vi "Main Test Panel.vi"() -> ()   [LabVIEW 2013]
uses:
  Controls/DAQ Cluster.ctl
  <vilib>/DAQmx/create/channels.llb/DAQmx Create Channel (AI-Voltage-Basic).vi
panel:
  in  "Daq Clust 2":T2={"Save"=FALSE, "DAQ Cluster"={"PSI Channel"="Dev1/ai9", "TC Channel"="Dev1/ai10", "PSI Offset"=0.555, "PSI Scale"=3000.0, "TC Offset"=1.028, "TC Scale"=144.0}, "Cancel"=FALSE}
  in  "Start Averaging":bool
  in  "Time and Date":string
  out "DAQ On?":bool
  in  "Sim Cluster":T3 {"Temp" scale=0.0..35.0; "PSI" scale=0.0..20000.0}
  in  "Print to PDF":bool
  in  "Clear Graph":bool
  in  "DAQ Stop":bool
  in  "DAQ Start":bool
  in  "Test Duration (mins)":i32
  in  "Pressure (PSI)":i32
  in  "Test Temperature (°C)":i32
  in  "Tech Initials":string
  in  "Customer":string
  in  "Proof Test\nPressure (PSI)":i32
  in  "Time @ Proof\nPressure (mins)":i32=30
  in  "Max Working\nPressure (PSI)":i32
  in  "Serial #":string
  in  "Part Desc.":string
  in  "Part #":string
  out "Pressure Graph":dbl[][](graph)
  in  "Test Result":string
  # "Pressure Certificate"
  # "982 North 675 West\nNorth Salt Lake, UT 84054"
  # "Test Information"
  # "Test Results"
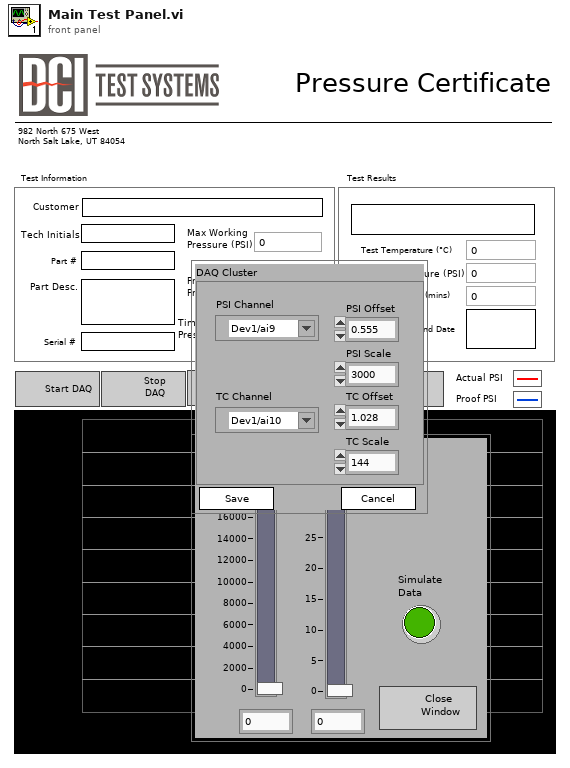
[diagram p1: front panel]
types:
  T1 = typedef "DAQ Cluster.ctl" = cluster{"PSI Channel":tag, "TC Channel":tag, "PSI Offset":dbl, "PSI Scale":dbl, "TC Offset":dbl, "TC Scale":dbl}
  T2 = cluster{"Save":bool, "DAQ Cluster":T1, "Cancel":bool}
  T3 = cluster{"PSI":i32, "Temp":i32, "Simulate\nData":bool, "Close Sim":bool}
  T4 = enum16{"open", "replace", "create", "open or create", "replace or create", "replace or create with confirmation"}
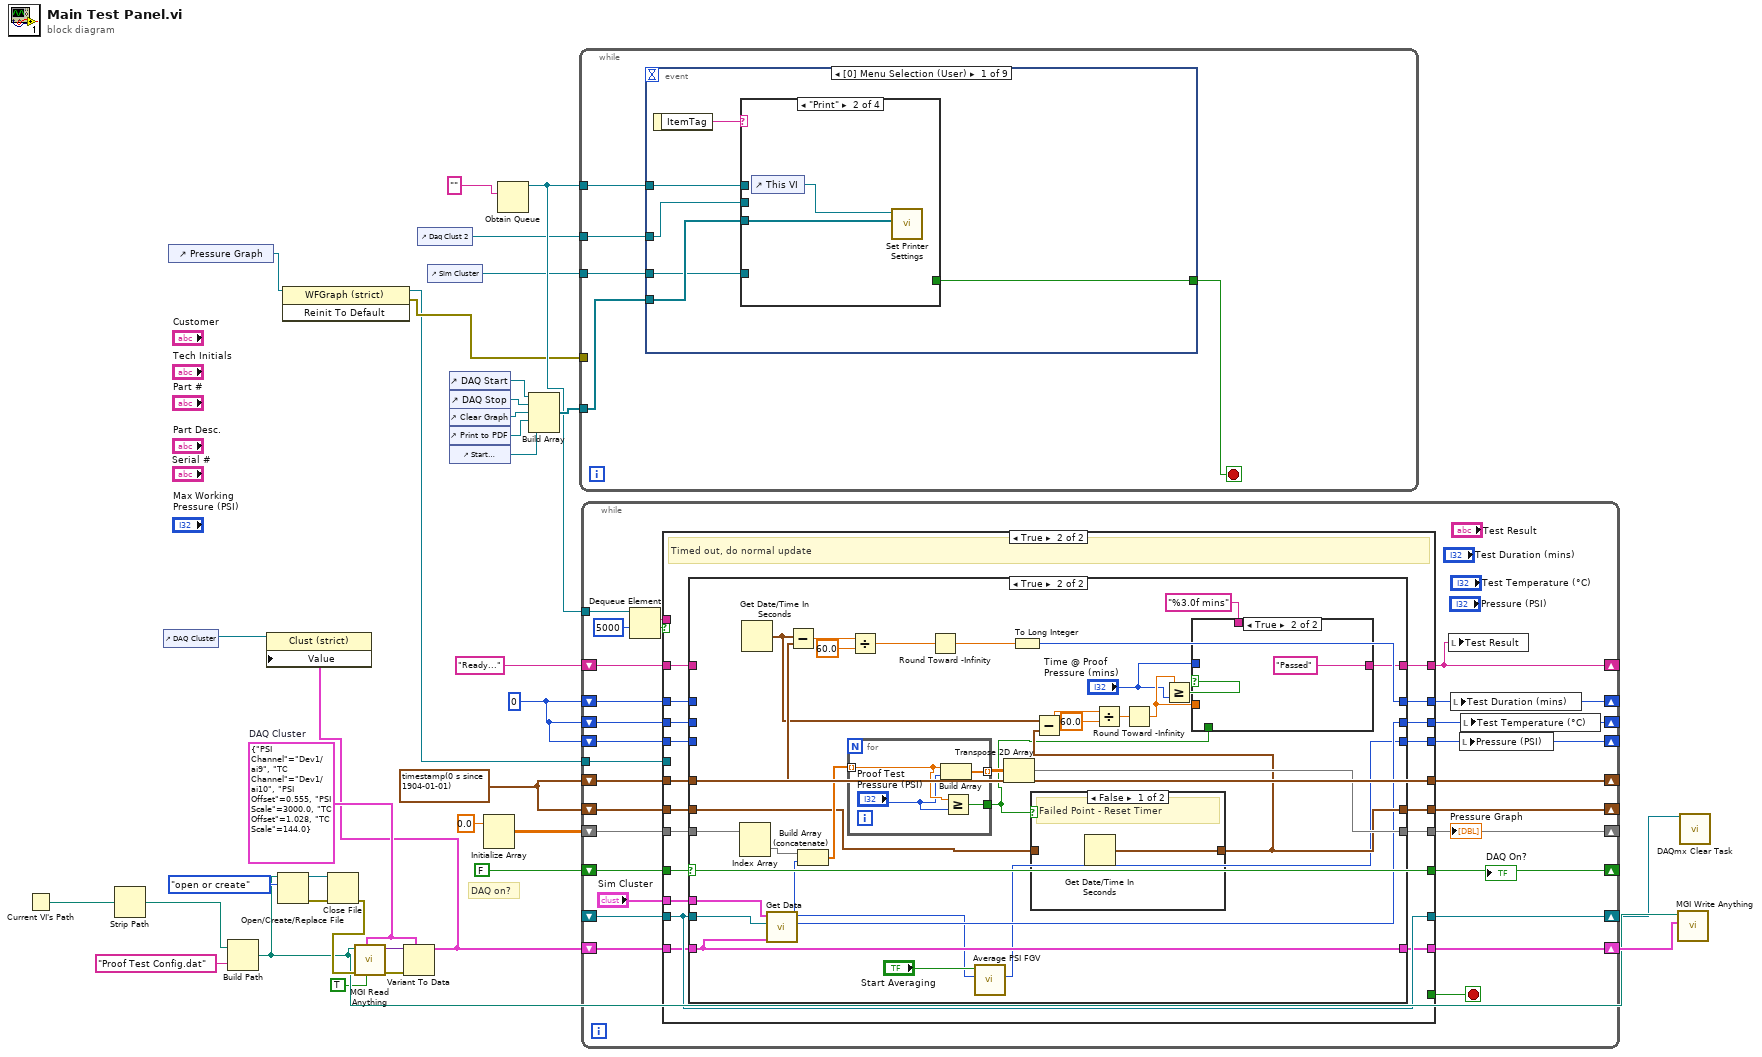
[diagram p0: block diagram]
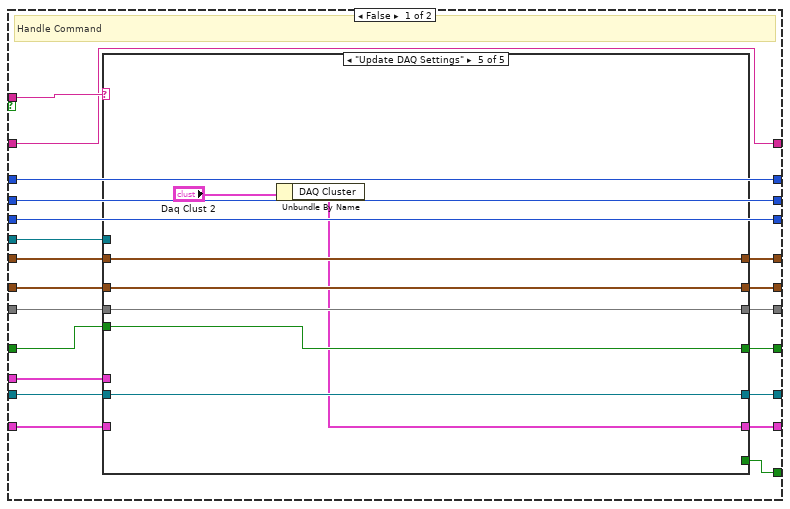
[diagram p2: hidden frame]
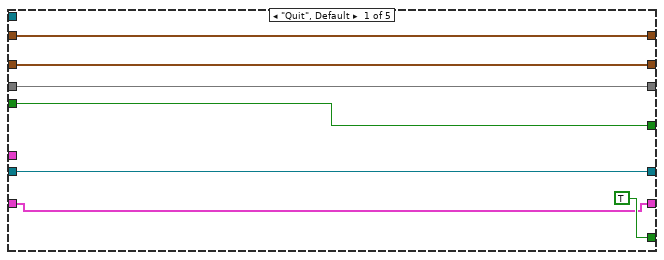
[diagram p3: hidden frame]
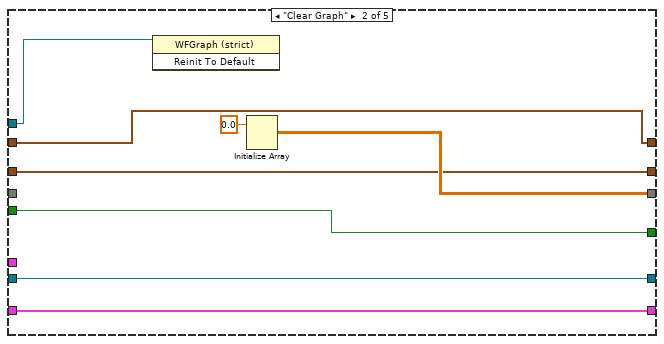
[diagram p4: hidden frame]
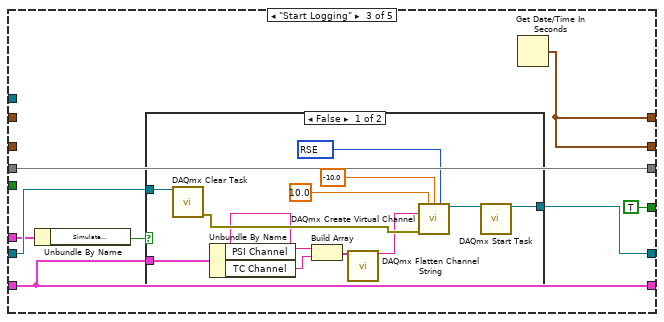
[diagram p5: hidden frame]
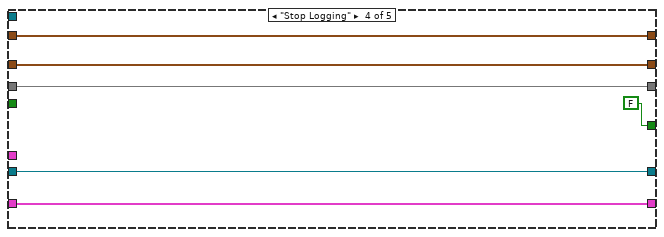
[diagram p7: hidden frame]
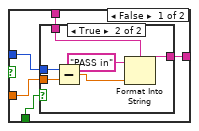
[diagram p9: hidden frame]
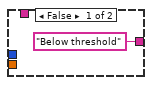
[diagram p10: hidden frame]
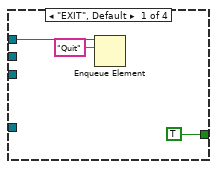
[diagram p12: hidden frame]
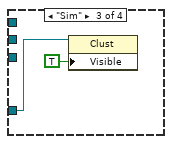
[diagram p13: hidden frame]
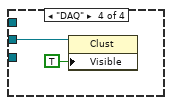
[diagram p14: hidden frame]
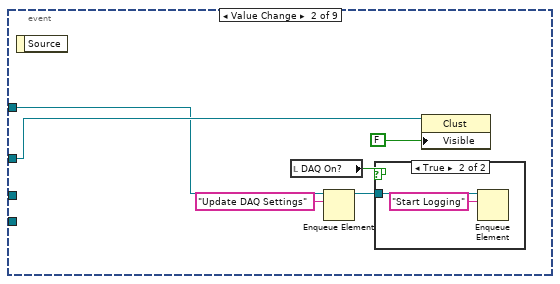
[diagram p15: hidden frame]
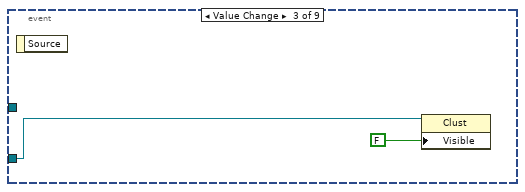
[diagram p17: hidden frame]
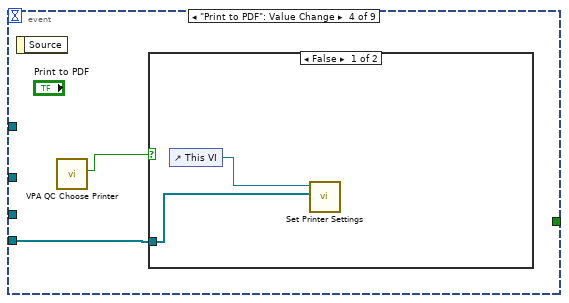
[diagram p18: hidden frame]
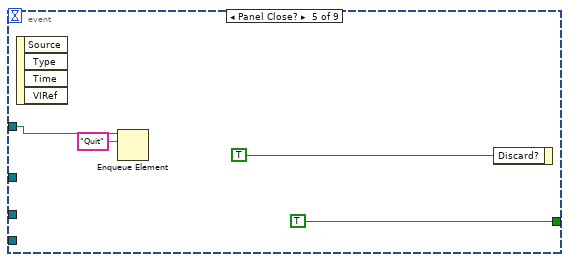
[diagram p20: hidden frame]
diagram:
  w10 = T1 {"PSI Channel"="Dev1/ai9", "TC Channel"="Dev1/ai10", "PSI Offset"=0.555, "PSI Scale"=3000.0, "TC Offset"=1.028, "TC Scale"=144.0}  # DAQ Cluster
  w21 = timestamp(0 s since 1904-01-01)
  w23 = 0 ("Test Duration (mins)")
  # "DAQ on?"
  n1 = Current VI's Path() -> (path=w16:path)
  n2 = Strip Path(path=w16) -> (stripped path=w5:path)  [unwired: 1 out]
  n3 = control-ref of="DAQ Cluster"() -> (w4:refnum<vi>)
  n4 = control-ref of="Pressure Graph"() -> (w28:refnum<vi>)
  n5 = Build Path(base path=w5, name or relative path="Proof Test Config.dat") -> (appended path=w8:path)
  n6 = Open/Create/Replace File(file path (use dialog)=w8, operation (0:open)=T4."open or create") -> (refnum out=w13:refnum<file>, error out=w12:errorcluster)  [unwired: 4 in, 1 out]
  n7 = invoke class="WFGraph (strict)" method="Reinit To Default"(reference=w28) -> (reference out=w19:refnum<vi>, error out=w25:errorcluster)  [unwired: 2 in, 1 out]
  n8 = Close File(refnum=w13, error in=w12) -> (error out=w11:errorcluster)  [unwired: 1 out]
  n9 = call <userlib>:"MGI Read Anything.vi"("Use Supplied (F: Use Default)"=TRUE, "Type of Anything"=w10, "Error In"=w11, "Path (dialog)"=w8) -> ("Error Out"=w18:errorcluster, "Anything"=w17:variant)  [unwired: 4 in, 2 out]
  n10 = Variant To Data(error in=w18, type=w10, Variant=w17) -> (data=w3:T1)  [unwired: 1 out]
  n11 = property class="Clust (strict)"(reference=w4, "Value"=w3) -> ()  [unwired: 1 in, 2 out]
  n12 = control-ref of="Daq Clust 2"() -> (w6:refnum<vi>)
  n13 = control-ref of="Sim Cluster"() -> (w20:refnum<vi>)
  n14 = control-ref of="DAQ Start"() -> (w35:refnum<vi>)
  n15 = control-ref of="DAQ Stop"() -> (w34:refnum<vi>)
  n16 = control-ref of="Clear Graph"() -> (w33:refnum<vi>)
  n17 = control-ref of="Print to PDF"() -> (w32:refnum<vi>)
  n18 = control-ref of="Start Averaging"() -> (w1:refnum<vi>)
  n19 = Initialize Array(0.0 ("element")) -> (w26:dbl[][])  [unwired: 2 in]
  n20 = Obtain Queue(element data type="") -> (queue out=w30:refnum<queue>)  [unwired: 4 in, 2 out]
  n21 = Build Array(w35, w34, w33, w32, w1) -> (w31:refnum<vi>[])
  n22 = while {
    tunnel: w31 -> [w39]
    tunnel: w30 -> [w38]
    tunnel: w25 -> [_]
    tunnel: w20 -> [w37]
    tunnel: w6 -> [w36]
    stop <- w40 stop-if-true
    n23 = event shown="[0] Menu Selection (User)" {
      selector: _ -> [_ _ _ _ _ _ _ _ _]
      dyn-events: _ -> [_ _ _ _ _ _ _ _ _]
      timeout: _ -> [_ _ _ _ _ _ _ _ _]
      tunnel: [w45 _ _ _ TRUE _ _ _ _] -> w40
      tunnel: w39 -> [w44 _ _ w66 _ _ _ _ _]
      tunnel: w38 -> [w43 w59 _ _ w71 w75 w82 w84 _]
      tunnel: w37 -> [w42 _ _ _ _ _ _ _ w86]
      tunnel: w36 -> [w41 w61 w65 _ _ _ _ _ _]
      event Menu Selection (User) {
        n24 = event-data() -> ("ItemTag"=w46:string)  [unwired: 1 in]
        n25 = case shown="\"Print\"" w46 {
          tunnel: [TRUE _ _ _] -> w45
          tunnel: w44 -> [_ w50 _ _]
          tunnel: w43 -> [w48 _ _ _]
          tunnel: w42 -> [_ _ w53 _]
          tunnel: w41 -> [_ _ _ w54]
          frame "EXIT", Default {
            n26 = Enqueue Element(queue=w48, element="Quit") -> ()  [unwired: 2 in, 3 out]
          }
          frame "Print" {
            n27 = control-ref of="This VI"() -> (w51:refnum<vi>)
            n28 = call "Set Printer Settings.vi"("Array"=w50, "VI in"=w51) -> ()  [unwired: 10 in]
          }
          frame "Sim" {
            n29 = property class="Clust"(reference=w53, "Visible"=TRUE) -> ()  [unwired: 1 in, 2 out]
          }
          frame "DAQ" {
            n30 = property class="Clust"(reference=w54, "Visible"=TRUE) -> ()  [unwired: 1 in, 2 out]
          }
        }
      }
      event "Daq Clust 2.Save": Value Change {
        n31 = event-data() -> ()  [unwired: 1 in, 1 out]
        n32 = local read "DAQ On?"() -> (w56:bool)
        n33 = Enqueue Element(queue=w59, element="Update DAQ Settings") -> (queue out=w57:refnum<queue>)  [unwired: 2 in, 2 out]
        n34 = case shown="True" w56 {
          tunnel: w57 -> [_ w63]
          frame False {
          }
          frame True {
            n35 = Enqueue Element(queue=w63, element="Start Logging") -> ()  [unwired: 2 in, 3 out]
          }
        }
        n36 = property class="Clust"(reference=w61, "Visible"=FALSE) -> ()  [unwired: 1 in, 2 out]
      }
      event "Daq Clust 2.Cancel": Value Change {
        n37 = event-data() -> ()  [unwired: 1 in, 1 out]
        n38 = property class="Clust"(reference=w65, "Visible"=FALSE) -> ()  [unwired: 1 in, 2 out]
      }
      event "Print to PDF": Value Change {
        n39 = event-data() -> ()  [unwired: 1 in, 1 out]
        n40 = call "VPA QC Choose Printer.vi"() -> ("Cancelled"=w67:bool)  [unwired: 11 in]
        n41 = case shown="False" w67 {
          tunnel: w66 -> [w69 _]
          frame False {
            n42 = control-ref of="This VI"() -> (w68:refnum<vi>)
            n43 = call "Set Printer Settings.vi"("Array"=w69, "VI in"=w68) -> ()  [unwired: 10 in]
          }
          frame True {
          }
        }
      }
      event Panel Close? {
        n44 = event-data() -> ()  [unwired: 1 in, 4 out]
        n45 = Enqueue Element(queue=w71, element="Quit") -> ()  [unwired: 2 in, 3 out]
        n46 = event-data("Discard?"=TRUE) -> ()  [unwired: 1 in, 1 out]
      }
      event "Clear Graph": Value Change {
        n47 = event-data() -> ()  [unwired: 1 in, 1 out]
        n48 = Enqueue Element(queue=w75, element="Clear Graph") -> ()  [unwired: 2 in, 3 out]
      }
      event "DAQ Start": Value Change {
        n49 = event-data() -> ()  [unwired: 1 in, 1 out]
        n50 = Enqueue Element(queue=w82, element="Start Logging") -> ()  [unwired: 2 in, 3 out]
        n51 = Get Date/Time In Seconds() -> (seconds since 1Jan1904=w80:timestamp)
        n52 = Get Date/Time String(seconds (now)=w80) -> (date string=w77:string, time string=w79:string)  [unwired: 2 in]
        n53 = Concatenate Strings(w79, "\n" ("string"), w77) -> (w76:string)
        n54 = local write "Time and Date"(w76) -> ()
      }
      event "DAQ Stop": Value Change {
        n55 = event-data() -> ()  [unwired: 1 in, 1 out]
        n56 = Enqueue Element(queue=w84, element="Stop Logging") -> ()  [unwired: 2 in, 3 out]
      }
      event "Sim Cluster.Close Sim": Value Change {
        n57 = event-data() -> ()  [unwired: 1 in, 6 out]
        n58 = property class="Clust"(reference=w86, "Visible"=FALSE) -> ()  [unwired: 1 in, 2 out]
      }
    }
  }
  n59 = while {
    tunnel: w30 -> [w113]
    shift-right: [w105] -> _
    shift-left: w26 -> [w108]
    shift-right: [w106] -> _
    shift-left: FALSE -> [w107]
    shift-right: [w91] -> _
    shift-left: "Ready..." -> [w104]
    shift-right: [w89] -> _
    shift-left: w23 -> [w103]
    shift-right: [w90] -> _
    shift-left: w23 -> [w102]
    shift-right: [w88] -> _
    shift-left: w23 -> [w101]
    shift-right: [w100] -> _
    shift-left: w21 -> [w99]
    shift-right: [w97] -> _
    shift-left: w21 -> [w98]
    tunnel: w19 -> [w96]
    shift-right: [w95] -> w2
    shift-left: _ -> [w94]
    shift-right: [w92] -> w9
    shift-left: w3 -> [w93]
    stop <- w109 stop-if-true
    n60 = Dequeue Element(queue=w113, timeout in ms (-1)=5000) -> (element=w110:string, timed out?=w112:bool)  [unwired: 1 in, 2 out]
    n61 = case shown="True" w112 {
      tunnel: w110 -> [w133 _]
      tunnel: [w132 _] -> w109
      tunnel: w108 -> [w131 w197]
      tunnel: [w130 w195] -> w105
      tunnel: w107 -> [w129 w194]
      tunnel: [w128 w194] -> w106
      tunnel: w104 -> [w127 w190]
      tunnel: [w127 w188] -> w91
      tunnel: [w124 w199] -> w89
      tunnel: w103 -> [w124 w193]
      tunnel: [w123 w198] -> w90
      tunnel: w102 -> [w123 w191]
      tunnel: [w122 w196] -> w88
      tunnel: w101 -> [w122 w192]
      tunnel: [w126 w200] -> w100
      tunnel: w99 -> [w125 w200]
      tunnel: w98 -> [w120 w189]
      tunnel: [w121 w187] -> w97
      tunnel: w96 -> [w119 _]
      tunnel: [w118 w186] -> w95
      tunnel: w94 -> [w117 w186]
      tunnel: w93 -> [w116 w185]
      tunnel: [w115 w184] -> w92
      tunnel: "Sim Cluster" -> [w114 w183]
      frame False {
        # "Handle Command"
        n62 = case shown="\"Update DAQ Settings\"" w133 {
          tunnel: [TRUE _ _ _ _] -> w132
          tunnel: w131 -> [w139 _ w156 w175 w178]
          tunnel: w119 -> [_ w147 _ _ _]
          tunnel: [w139 w146 w156 w175 w178] -> w130
          tunnel: w129 -> [w138 w145 _ _ w179]
          tunnel: [w138 w145 TRUE FALSE w179] -> w128
          tunnel: [w137 w144 w154 w173 w182] -> w126
          tunnel: w125 -> [w137 w144 _ w173 w182]
          tunnel: [w136 w143 w154 w172 w181] -> w121
          tunnel: w120 -> [w136 w143 _ w172 w181]
          tunnel: [w135 w142 w151 w171 w180] -> w118
          tunnel: w117 -> [w135 w142 w152 w171 w180]
          tunnel: w116 -> [w134 w141 w153 w170 _]
          tunnel: [w134 w141 w153 w170 w176] -> w115
          tunnel: w114 -> [_ _ w150 _ _]
          frame "Quit", Default {
          }
          frame "Clear Graph" {
            n63 = invoke class="WFGraph (strict)" method="Reinit To Default"(reference=w147) -> ()  [unwired: 2 in, 3 out]
            n64 = Initialize Array(0.0 ("element")) -> (w146:dbl[][])  [unwired: 2 in]
          }
          frame "Start Logging" {
            n65 = Unbundle By Name(w150) -> ("Simulate\nData"=w149:bool)
            n66 = case shown="False" w149 {
              tunnel: w153 -> [w165 _]
              tunnel: w152 -> [w163 w169]
              tunnel: [w161 w169] -> w151
              frame False {
                w168 = 10083 items=["default"=-1, "RSE"=10083, "NRSE"=10078, "Differential"=10106, "Pseudodifferential"=12529] ("input terminal configuration")
                n67 = call <vilib>:"DAQmx Clear Task.vi"("task in"=w163) -> ("error out"=w162:errorcluster)  [unwired: 14 in]
                n68 = Unbundle By Name(w165) -> ("PSI Channel"=w160:tag, "TC Channel"=w159:tag)
                n69 = Build Array(w160, w159) -> (w158:tag[])
                n70 = call <vilib>:"DAQmx Flatten Channel String.vi"("names in"=w158) -> ("names out"=w157:string)  [unwired: 13 in, 1 out]
                n71 = call-poly <vilib>:"DAQmx Create Virtual Channel.vi"("maximum value"=10.0, "minimum value"=-10.0, "input terminal configuration"=w168, "physical channels"=w157, "error in"=w162) -> ("task out"=w164:refnum<k21>)  [unwired: 9 in, 1 out]
                n72 = call <vilib>:"DAQmx Start Task.vi"("task/channels in"=w164) -> ("task out"=w161:refnum<k21>)  [unwired: 13 in, 1 out]
              }
              frame True {
              }
            }
            n73 = Get Date/Time In Seconds() -> (seconds since 1Jan1904=w154:timestamp)
          }
          frame "Stop Logging" {
          }
          frame "Update DAQ Settings" {
            n74 = Unbundle By Name("Daq Clust 2") -> ("DAQ Cluster"=w176:T1)
          }
        }
      }
      frame True {
        # "Timed out, do normal update"
        n75 = case shown="True" w194 {
          tunnel: w200 -> [_ w237]
          tunnel: [w207 w233] -> w199
          tunnel: [w204 w214] -> w198
          tunnel: w197 -> [w206 w232]
          tunnel: [w205 w210] -> w196
          tunnel: [w206 w228] -> w195
          tunnel: w193 -> [w207 _]
          tunnel: w192 -> [w205 _]
          tunnel: w191 -> [w204 _]
          tunnel: w190 -> [w203 _]
          tunnel: w189 -> [w202 w226]
          tunnel: [w203 w220] -> w188
          tunnel: [w202 w219] -> w187
          tunnel: w186 -> [_ w213]
          tunnel: w185 -> [w201 w212]
          tunnel: [w201 w212] -> w184
          tunnel: w183 -> [_ w209]
          frame False {
          }
          frame True {
            n76 = Index Array(array=w232) -> (element=w231:dbl[])  [unwired: 2 in]
            n77 = Get Date/Time In Seconds() -> (seconds since 1Jan1904=w225:timestamp)
            n78 = call "Get Data.vi"("DAQ Cluster"=w212, "DAQ Channels In"=w213, "Sim Cluster"=w209) -> ("Temp"=w214:i32, "PSI"=w208:i32)  [unwired: 7 in]
            n79 = Subtract(x=w225, y=w237) -> (x-y=w236:dbl)
            n80 = Build Array (concatenate)(w231, w208) -> (w230:dbl[])
            n81 = for {
              tunnel: w230 -> [w255] mode=indexing
              tunnel: [w256] -> w229 mode=indexing
              tunnel: [w253] -> w215
              n82 = Build Array(w255, "Proof Test\nPressure (PSI)") -> (w256:dbl[])
              n83 = Greater Or Equal?(x=w255, y="Proof Test\nPressure (PSI)") -> (x >= y?=w253:bool)
            }
            n84 = Divide(x=w236, y=60.0) -> (x/y=w234:dbl)
            n85 = Round Toward -Infinity(1:w234) -> (0:w227:dbl)
            n86 = call "Average PSI FGV.vi"("Current Pressure."=w208, "Average On?"="Start Averaging") -> ("Average Pressure"=w210:i32)  [unwired: 9 in]
            n87 = Transpose 2D Array(2D array=w229) -> (transposed array=w228:dbl[][])
            n88 = To Long Integer(number=w227) -> (32bit integer=w233:i32)
            n89 = case shown="False" w215 {
              tunnel: w226 -> [_ w252]
              tunnel: [w251 w252] -> w219
              frame False {
                # "Failed Point - Reset Timer"
                n90 = Get Date/Time In Seconds() -> (seconds since 1Jan1904=w251:timestamp)
              }
              frame True {
              }
            }
            n91 = Subtract(x=w225, y=w219) -> (x-y=w222:dbl)
            n92 = Divide(x=w222, y=60.0) -> (x/y=w224:dbl)
            n93 = Round Toward -Infinity(1:w224) -> (0:w218:dbl)
            n94 = Greater Or Equal?(x=w218, y="Time @ Proof\nPressure (mins)") -> (x >= y?=w221:bool)
            n95 = case shown="True" w221 {
              tunnel: [w242 "Passed"] -> w220
              tunnel: w218 -> [w240 _]
              tunnel: "Time @ Proof\nPressure (mins)" -> [w241 _]
              tunnel: "%3.0f mins" ("format string") -> [w239 _]
              tunnel: w215 -> [w238 _]
              frame False {
                n96 = case shown="True" w238 {
                  tunnel: ["Below threshold" w249] -> w242
                  tunnel: w241 -> [_ w248]
                  tunnel: w240 -> [_ w247]
                  tunnel: w239 -> [_ w245]
                  frame False {
                  }
                  frame True {
                    n97 = Subtract(x=w248, y=w247) -> (x-y=w246:dbl)
                    n98 = Format Into String(format string=w245, initial string="PASS in", w246) -> (resulting string=w249:string)  [unwired: 1 in, 1 out]
                  }
                }
              }
              frame True {
              }
            }
          }
        }
      }
    }
    "Pressure Graph" <- w105
    "DAQ On?" <- w106
    n99 = local write "Test Result"(w91) -> ()
    n100 = local write "Test Duration (mins)"(w89) -> ()
    n101 = local write "Pressure (PSI)"(w88) -> ()
    n102 = local write "Test Temperature (°C)"(w90) -> ()
  }
  n103 = call <userlib>:"MGI Write Anything.vi"("Anything"=w9, "Path (dialog)"=w8) -> ()  [unwired: 7 in, 3 out]
  n104 = call <vilib>:"DAQmx Clear Task.vi"("task in"=w2) -> ()  [unwired: 14 in, 1 out]
